vi "micron_start.vi"(8 "error in":errorcluster, 11 "Micron config":T1) -> (0 "error out":errorcluster)   [LabVIEW 2014]
uses:
  micron_config.ctl
  manipulator/squiggle/Host/i2c_interface.ctl
  manipulator/squiggle/Host/fpga_reference.ctl
  testing/Micron params.ctl
  testing/stimulus.ctl
  testing/injection_point.ctl
  filtering/goal_loop_parms.ctl
  testing/mode_conrols.ctl
  testing/manipulator_cal.ctl
  asap/labview/testing/probe_calibration.ctl
  host/network_params.ctl
  cancellation/sq_control_params.ctl
  cancellation/decoupled_gain.ctl
  cancellation/estimation_controls.ctl
  asap/labview/initialization/globals.vi
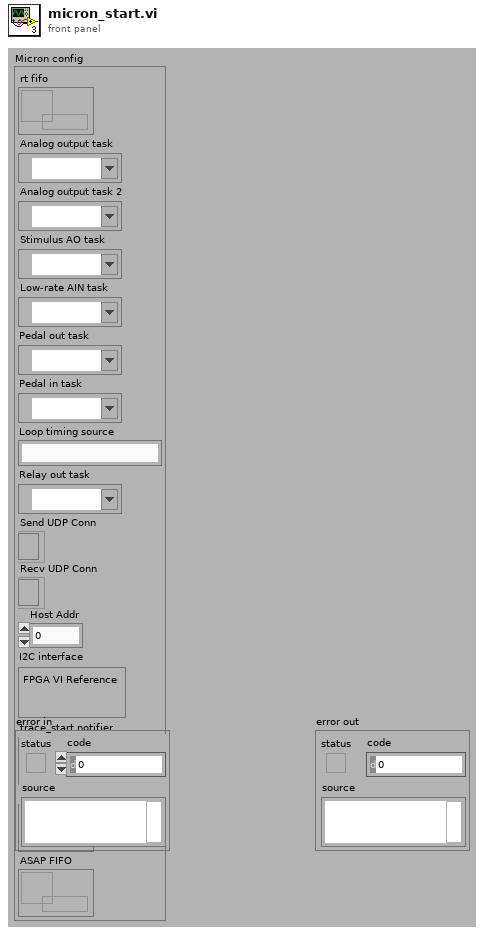
[diagram p1: front panel]
types:
  T1 = typedef "micron_config.ctl" = cluster{"rt fifo":refnum<k33>, "Analog output task":refnum<k21>, "Analog output task 2":refnum<k21>, "Stimulus AO task":refnum<k21>, "Low-rate AIN task":refnum<k21>, "Pedal out task":refnum<k21>, "Pedal in task":refnum<k21>, "Loop timing source":string, "Relay out task":refnum<k21>, "Send UDP Conn":refnum<k16>, "Recv UDP Conn":refnum<k16>, "Host Addr":u32, "I2C interface":T2, "trace_start notifier":refnum<notifier>, "trace_done notifier":refnum<notifier>, "ASAP FIFO":refnum<k33>}
  T2 = typedef "i2c_interface.ctl" = cluster{"FPGA VI Reference":T3}
  T3 = typedef "fpga_reference.ctl" = refnum<k20>
  T4 = enum16{"ASAP/Trigger", "ASAP/Finder", "ASAP/Micron", "ASAP/Micron 2", "Micron 6DOF"}
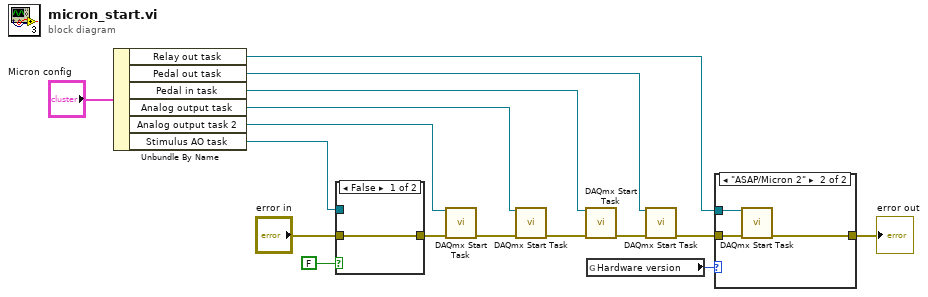
[diagram p0: block diagram]
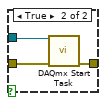
[diagram p2: hidden frame]
diagram:
  n1 = Unbundle By Name("Micron config") -> ("Relay out task"=w5:refnum<k21>, "Pedal out task"=w3:refnum<k21>, "Pedal in task"=w10:refnum<k21>, "Analog output task"=w13:refnum<k21>, "Analog output task 2"=w14:refnum<k21>, "Stimulus AO task"=w15:refnum<k21>)
  n2 = case shown="False" FALSE {
    tunnel: w15 -> [_ w20]
    tunnel: [w17 w19] -> w12
    tunnel: "error in" -> [w17 w18]
    frame False {
    }
    frame True {
      n3 = call <vilib>:"DAQmx Start Task.vi"("task/channels in"=w20, "error in"=w18) -> ("error out"=w19:errorcluster)  [unwired: 13 out]
    }
  }
  n4 = call <vilib>:"DAQmx Start Task.vi"("task/channels in"=w14, "error in"=w12) -> ("error out"=w11:errorcluster)  [unwired: 13 out]
  n5 = call <vilib>:"DAQmx Start Task.vi"("task/channels in"=w13, "error in"=w11) -> ("error out"=w9:errorcluster)  [unwired: 13 out]
  n6 = call <vilib>:"DAQmx Start Task.vi"("task/channels in"=w10, "error in"=w9) -> ("error out"=w4:errorcluster)  [unwired: 13 out]
  n7 = global read "globals.vi" "Hardware version"() -> (w6:T4)
  n8 = call <vilib>:"DAQmx Start Task.vi"("task/channels in"=w3, "error in"=w4) -> ("error out"=w2:errorcluster)  [unwired: 13 out]
  n9 = case shown="\"ASAP/Micron 2\"" w6 {
    tunnel: w2 -> [w21 w24]
    tunnel: w5 -> [_ w23]
    tunnel: [w21 w22] -> w8
    frame "ASAP/Trigger", Default {
    }
    frame "ASAP/Micron 2" {
      n10 = call <vilib>:"DAQmx Start Task.vi"("task/channels in"=w23, "error in"=w24) -> ("error out"=w22:errorcluster)  [unwired: 13 out]
    }
  }
  "error out" <- w8
